vi "Copy.vi"(8 "error in":errorcluster, 10 "Image Dst Reference In":T1, 11 "Image Src Reference In":T1) -> (0 "error out":errorcluster, 3 "Image Dst Reference Out":T1)   [LabVIEW 2020, in "OpenLvVision_Image.lvlib" / "Management.lvlib"]
doc: "Creates an independent duplicate of an image, including its pixel data, dimensions, and metadata. Modifications to the copy do not affect the original."
uses:
  Management.lvlib
  TypeDef/Image.ctl
  DataAccess/DataAccess.lvlib
  DLLs/OLV_VisionCore_AVX2_X64.dll
  DLLs/OLV_VisionCore_AVX2_X86.dll
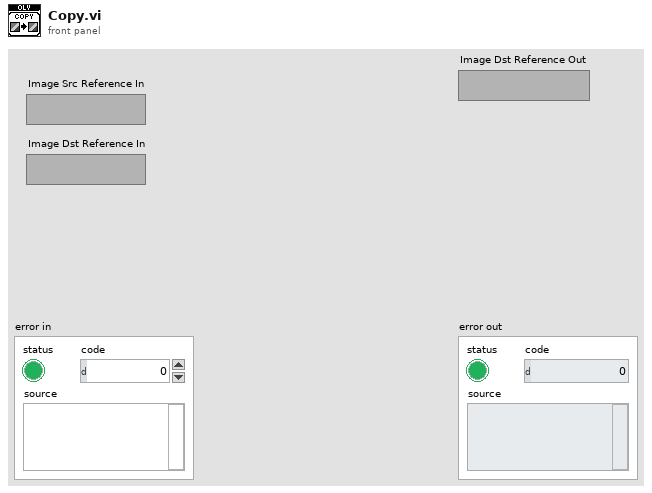
[diagram p1: front panel]
types:
  T1 = typedef "OpenLvVision_Image.lvlib/Management.lvlib/Image.ctl" = refnum<image>
  T2 = typedef "OpenLvVision_Image.lvlib/DataAccess.lvlib/PixelPointer.ctl" = cluster{"Image Border Size":i32, "Pixel Pointer":u64, "LineWidth":i32, "PixelSize_Bytes":i32, "TransferMaxSize":i32}
  T3 = typedef "OpenLvVision_Image.lvlib/Management.lvlib/ImageType.ctl" = enum16{"Mono U8", "Mono U16", "Mono I16", "Mono SGL", "Color U32", "Color U64", "Complex CSG"}
  T4 = typedef "IMAQ Image.ctl" = refnum<image>
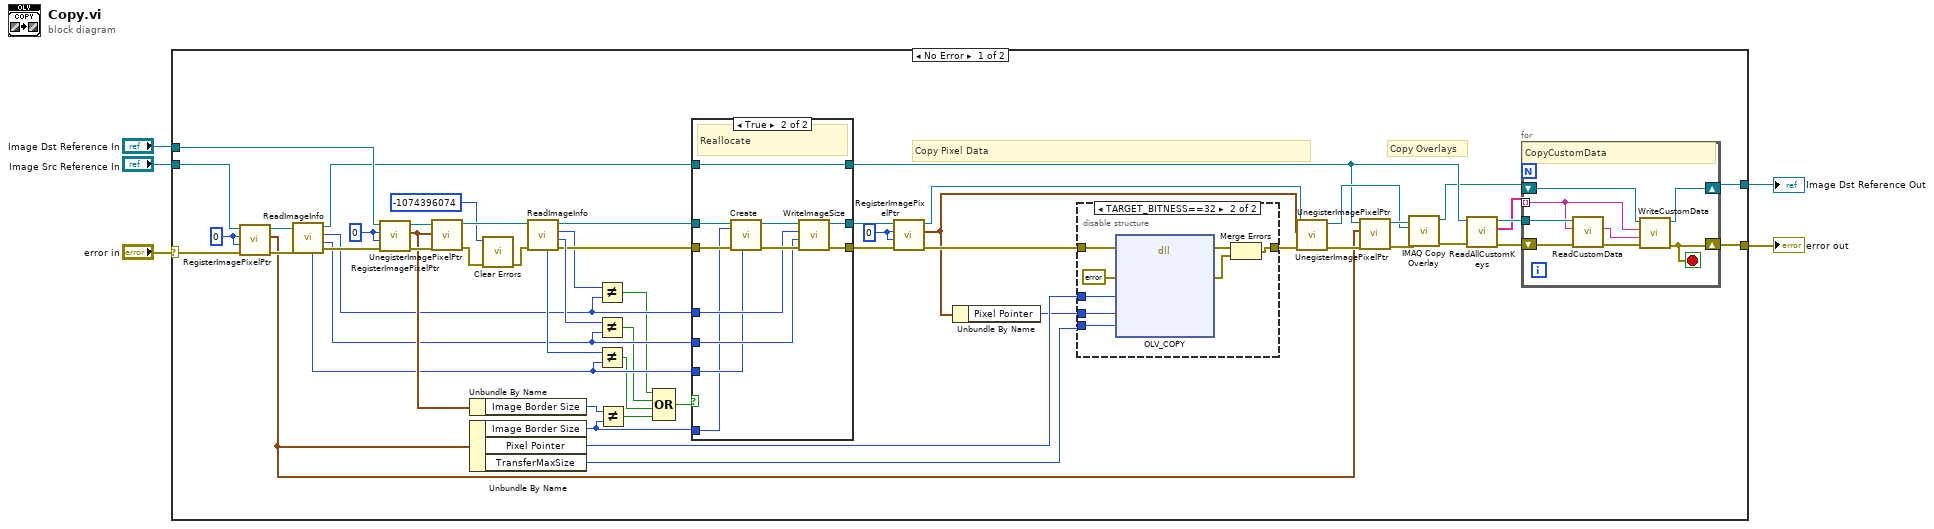
[diagram p0: block diagram]
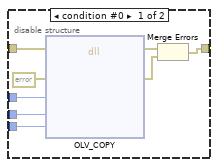
[diagram p2: hidden frame]
diagram:
  n1 = case shown="No Error" "error in" {
    selector: "error in" -> [w59 w98]
    tunnel: "Image Src Reference In" -> [w58 _]
    tunnel: "Image Dst Reference In" -> [w57 w99]
    tunnel: [w13 w99] -> w2
    tunnel: [w16 w98] -> w1
    frame No Error {
      w31 = 0
      w52 = 0
      w53 = 0
      # "Copy Pixel Data"
      # "Copy Overlays"
      n2 = call "RegisterImagePixelPtr.vi"("error in"=w59, "Y Coordinate"=w53, "X Coordinate"=w53, "Image Reference In"=w58) -> ("error out"=w55:errorcluster, "PixelPointer"=w12:T2, "Image Reference Out"=w56:T1)  [unwired: 5 in]
      n3 = call "ReadImageInfo.vi"("error in"=w55, "Image Reference In"=w56) -> ("error out"=w54:errorcluster, "Height"=w36:i32, "Width"=w37:i32, "Image Reference Out"=w40:T1, "Image Type"=w35:T3)  [unwired: 4 in, 1 out]
      n4 = call "RegisterImagePixelPtr.vi"("error in"=w54, "Y Coordinate"=w52, "X Coordinate"=w52, "Image Reference In"=w57) -> ("error out"=w50:errorcluster, "PixelPointer"=w49:T2, "Image Reference Out"=w51:T1)  [unwired: 5 in]
      n5 = call "UnegisterImagePixelPtr.vi"("error in"=w50, "PixelPointer"=w49, "Image Reference In"=w51) -> ("error out"=w8:errorcluster, "Image Reference Out"=w48:T1)  [unwired: 7 in]
      n6 = Unbundle By Name(w49) -> ("Image Border Size"=w47:i32)
      n7 = Unbundle By Name(w12) -> ("Image Border Size"=w38:i32, "Pixel Pointer"=w23:u64, "TransferMaxSize"=w9:i32)
      n8 = call <vilib>:"Clear Errors.vi"("error in (no error)"=w8, "specific error code to clear (0: all)"=-1074396074) -> ("error out"=w7:errorcluster)  [unwired: 4 in, 1 out]
      n9 = call "ReadImageInfo.vi"("error in"=w7, "Image Reference In"=w48) -> ("error out"=w41:errorcluster, "Height"=w46:i32, "Width"=w39:i32, "Image Reference Out"=w42:T1, "Image Type"=w45:T3)  [unwired: 4 in, 1 out]
      n10 = Not Equal?(x=w39, y=w37) -> (x != y?=w32:bool)
      n11 = Not Equal?(x=w46, y=w36) -> (x != y?=w33:bool)
      n12 = Not Equal?(x=w45, y=w35) -> (x != y?=w34:bool)
      n13 = Not Equal?(x=w47, y=w38) -> (x != y?=w44:bool)
      n14 = Compound Arithmetic op=OR(w32, w33, w34, w44) -> (w43:bool)
      n15 = case shown="True" w43 {
        tunnel: w42 -> [w77 w87]
        tunnel: w41 -> [w78 w86]
        tunnel: w40 -> [w76 w81]
        tunnel: w38 -> [_ w82]
        tunnel: w37 -> [_ w85]
        tunnel: w36 -> [_ w84]
        tunnel: w35 -> [_ w83]
        tunnel: [w76 w81] -> w15
        tunnel: [w77 w80] -> w30
        tunnel: [w78 w79] -> w29
        frame False {
        }
        frame True {
          # "Reallocate"
          n16 = call "Create.vi"("Image Type"=w83, "Border"=w82, "error in"=w86, "Image Name"=w87) -> ("error out"=w88:errorcluster, "Image Reference Out"=w89:T1)  [unwired: 6 in]
          n17 = call "WriteImageSize.vi"("error in"=w88, "Height"=w84, "Width"=w85, "Image Reference In"=w89) -> ("error out"=w79:errorcluster, "Image Reference Out"=w80:T1)  [unwired: 6 in]
        }
      }
      n18 = call "RegisterImagePixelPtr.vi"("error in"=w29, "Y Coordinate"=w31, "X Coordinate"=w31, "Image Reference In"=w30) -> ("error out"=w28:errorcluster, "PixelPointer"=w24:T2, "Image Reference Out"=w27:T1)  [unwired: 5 in]
      n19 = Unbundle By Name(w24) -> ("Pixel Pointer"=w22:u64)
      n20 = disable-structure shown="TARGET_BITNESS==32" {
        disable-tunnel: w28 -> [w67 w75]
        disable-tunnel: [w61 w70] -> w25
        disable-tunnel: w23 -> [w66 w74]
        disable-tunnel: w22 -> [w65 w73]
        disable-tunnel: w9 -> [w64 w72]
        frame condition #0 {
          n21 = dll-call lib="C:/Users/lukas/Downloads/OpenLvVision_Image/SourceCode/DLLs/OLV_VisionCore_AVX2_X64.dll" fn="OLV_COPY"(error in=w67, "Error"=errorcluster {"status"=FALSE, "code"=0, "source"=""} ("error out"), "SrcPtr"=w66, "DstPtr"=w65, "Bytes"=w64) -> (error out=w63:errorcluster, "Error"=w62:errorcluster)  [unwired: 6 in, 1 out]
          n22 = Merge Errors(w63, w62) -> (w61:errorcluster)
        }
        frame condition #1 (active) {
          n23 = dll-call lib="C:/Users/lukas/Downloads/OpenLvVision_Image/SourceCode/DLLs/OLV_VisionCore_AVX2_X86.dll" fn="OLV_COPY"(error in=w75, "Error"=errorcluster {"status"=FALSE, "code"=0, "source"=""} ("error out"), "SrcPtr"=w74, "DstPtr"=w73, "Bytes"=w72) -> (error out=w71:errorcluster, "Error"=w69:errorcluster)  [unwired: 6 in, 1 out]
          n24 = Merge Errors(w71, w69) -> (w70:errorcluster)
        }
      }
      n25 = call "UnegisterImagePixelPtr.vi"("error in"=w25, "PixelPointer"=w24, "Image Reference In"=w27) -> ("error out"=w26:errorcluster, "Image Reference Out"=w19:T1)  [unwired: 7 in]
      n26 = call "UnegisterImagePixelPtr.vi"("error in"=w26, "PixelPointer"=w12, "Image Reference In"=w15) -> ("error out"=w21:errorcluster, "Image Reference Out"=w20:T1)  [unwired: 7 in]
      n27 = call "IMAQ Copy Overlay"("error in (no error)"=w21, "Image Dst"=w19, "Image Src"=w20) -> ("error out"=w18:errorcluster, "Image Dst Out"=w14:T4)  [unwired: 7 in]
      n28 = call "ReadAllCustomKeys.vi"("error in"=w18, "Image Reference In"=w15) -> ("error out"=w17:errorcluster, "Keys"=w10:string[], "Image Reference Out"=w11:T1)  [unwired: 6 in, 1 out]
      n29 = for {
        shift-right: [w90] -> w16
        shift-left: w17 -> [w97]
        shift-right: [w94] -> w13
        shift-left: w14 -> [w93]
        tunnel: w11 -> [w95]
        tunnel: w10 -> [w91] mode=indexing
        stop <- w90 stop-if-true
        # "CopyCustomData"
        n30 = call "ReadCustomData.vi"("error in"=w97, "Key"=w91, "Image Reference In"=w95) -> ("error out"=w96:errorcluster, "Data"=w92:string)  [unwired: 6 in, 1 out]
        n31 = call "WriteCustomData.vi"("error in"=w96, "Data"=w92, "Key"=w91, "Image Reference In"=w93) -> ("error out"=w90:errorcluster, "Image Reference Out"=w94:T1)  [unwired: 6 in]
      }
    }
    frame Error {
    }
  }
  "error out" <- w1
  "Image Dst Reference Out" <- w2
